vi "NanoScan Test Panel.vi"() -> ()   [LabVIEW 2020]
uses:
  <vilib>/Instr/_visa.llb/VISA Configure Serial Port (Instr).vi
panel:
  out "Device Info":string
  out "Cmd Success":bool
  out "Connected":bool
  out "Waiting for Reply":bool
  out "Last Error":errorcluster
  out "Command History":string
  out "Reply":string
  in  "Command":string
  in  "Quit":bool
  in  "COM Port":refnum<visa-resource-name>="COM4"
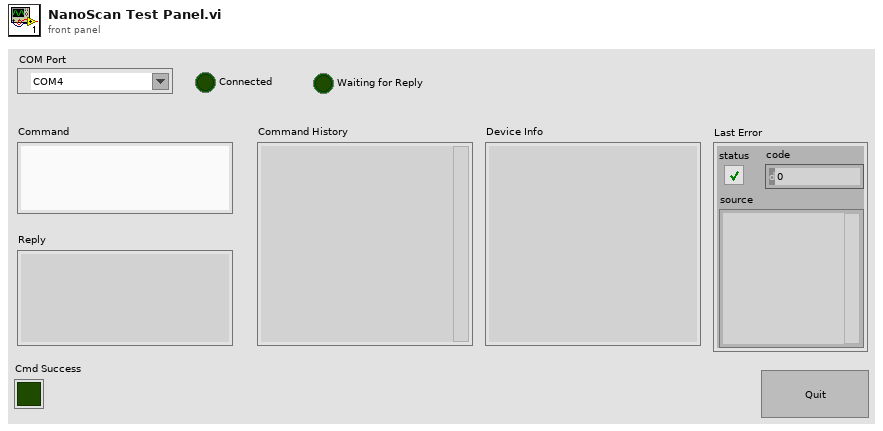
[diagram p1: front panel]
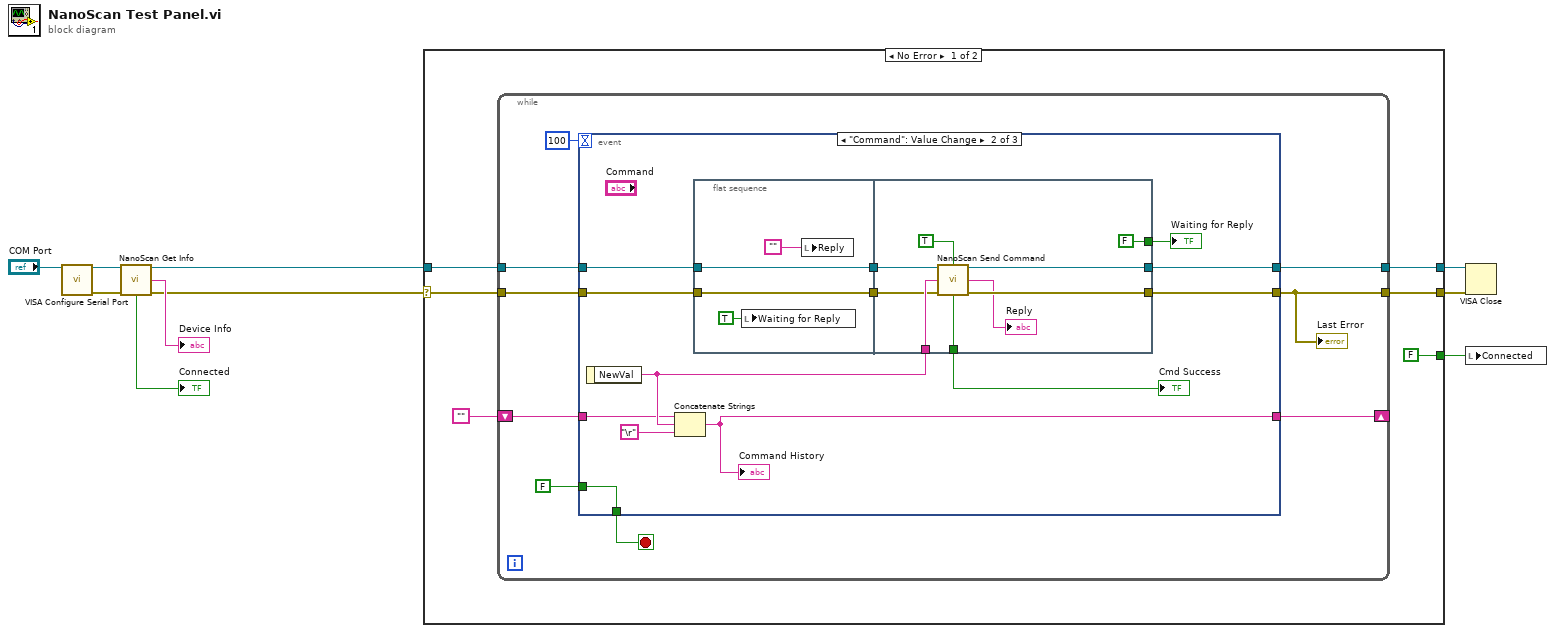
[diagram p0: block diagram]
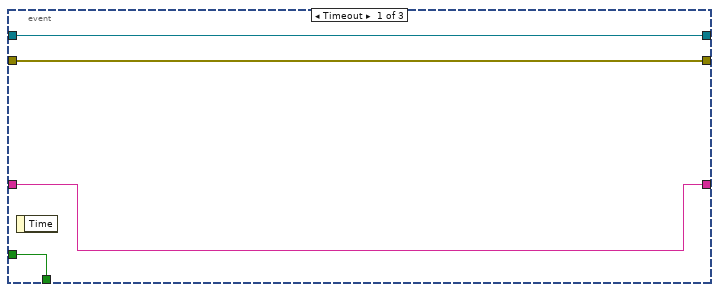
[diagram p2: hidden frame]
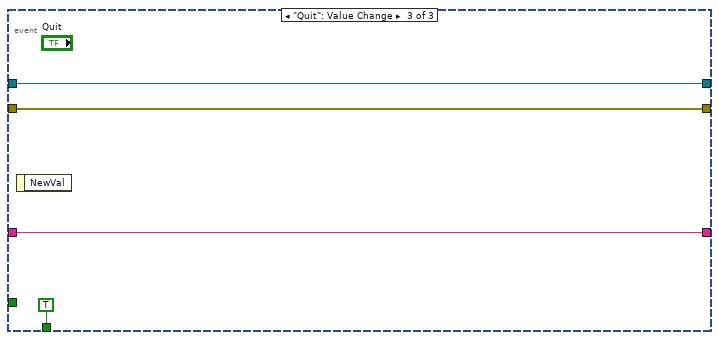
[diagram p3: hidden frame]
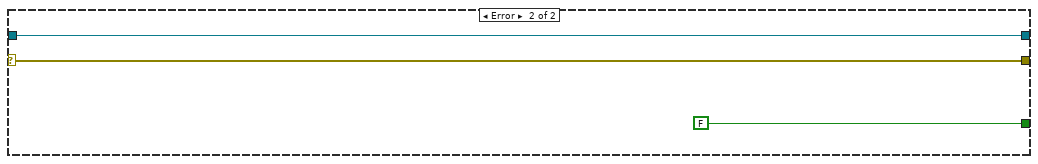
[diagram p4: hidden frame]
diagram:
  n1 = call-poly "VISA Configure Serial Port"("VISA resource name"="COM Port") -> ("VISA resource name out"=w6:refnum<visa-resource-name>, "error out"=w1:errorcluster)  [unwired: 13 in]
  n2 = call "NanoScan Get Info.vi"("VISA Ref"=w6, "Error In"=w1) -> ("VISA Ref Dup"=w5:refnum<visa-resource-name>, "Reply"=→"Device Info":string, "Connected"=→"Connected":bool, "Error Out"=w2:errorcluster)  [unwired: 10 in]
  n3 = case shown="No Error" w2 {
    selector: w2 -> [w15 w61]
    tunnel: w5 -> [w16 w62]
    tunnel: [w14 w62] -> w10
    tunnel: [w13 w61] -> w9
    tunnel: [FALSE FALSE] -> w8
    frame No Error {
      n4 = while {
        tunnel: w16 -> [w23]
        tunnel: w15 -> [w22]
        tunnel: [w21] -> w14
        tunnel: [w18] -> w13
        shift-right: [w19] -> _
        shift-left: "" -> [w20]
        stop <- w24 stop-if-true
        n5 = event shown="[1] \"Command\": Value Change" {
          selector: _ -> [_ _ _]
          dyn-events: _ -> [_ _ _]
          timeout: 100 -> [_ _ _]
          tunnel: FALSE -> [w29 w42 _]
          tunnel: [w29 w42 TRUE] -> w24
          tunnel: w23 -> [w27 w41 w59]
          tunnel: w22 -> [w26 w40 w58]
          tunnel: [w27 w36 w59] -> w21
          tunnel: [w26 w37 w58] -> w18
          tunnel: w20 -> [w28 w33 w56]
          tunnel: [w28 w32 w56] -> w19
          event Timeout {
            n6 = event-data() -> ()  [unwired: 1 in, 1 out]
          }
          event "Command": Value Change {
            n7 = event-data() -> ("NewVal"=w35:string)  [unwired: 1 in]
            n8 = Concatenate Strings(w33, w35, "\r") -> (w32:string)
            "Command History" <- w32
            n9 = flat-sequence {
              tunnel: w40 -> [w45]
              tunnel: w41 -> [w46]
              tunnel: [w46] -> w39
              tunnel: [w45] -> w38
              tunnel: w35 -> [w54]
              tunnel: w39 -> [w55]
              tunnel: w38 -> [w53]
              tunnel: [w52] -> w37
              tunnel: [w51] -> w36
              tunnel: [FALSE] -> w31
              tunnel: [w48] -> w30
              frame #0 {
                n10 = local write "Waiting for Reply"(TRUE ("Waiting for Cmd")) -> ()
                n11 = local write "Reply"("") -> ()
              }
              frame #1 {
                n12 = call "NanoScan Send Command.vi"("VISA Ref"=w55, "Wait for Reply (T)"=TRUE, "Command"=w54, "Error In"=w53) -> ("VISA Ref Dup"=w51:refnum<visa-resource-name>, "Reply"=→"Reply":string, "Cmd Success"=w48:bool, "Error Out"=w52:errorcluster)  [unwired: 8 in]
              }
            }
            "Waiting for Reply" <- w31
            "Cmd Success" <- w30
          }
          event "Quit": Value Change {
            n13 = event-data() -> ()  [unwired: 1 in, 1 out]
          }
        }
        "Last Error" <- w18
      }
    }
    frame Error {
    }
  }
  n14 = VISA Close(VISA resource name=w10, error in (no error)=w9) -> ()  [unwired: 1 out]
  n15 = local write "Connected"(w8) -> ()
